vi "SquareFromCenter.vi"(6 "Distance":i32=10, 10 "Top":i32, 11 "Left":i32) -> (0 "Bottom":i32, 1 "Right":i32, 2 "Top 2":i32, 3 "Left 2":i32)   [LabVIEW 2014]
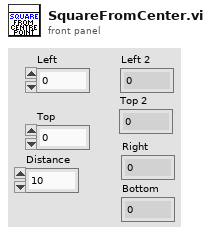
[diagram p1: front panel]
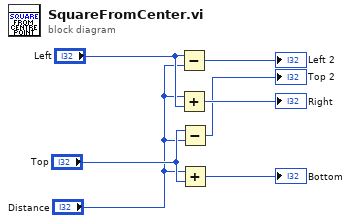
[diagram p0: block diagram]
diagram:
  n1 = Subtract(x="Left", y="Distance") -> (x-y=→"Left 2":i32)
  n2 = Add(x="Distance", y="Left") -> (x+y=→"Right":i32)
  n3 = Subtract(x="Top", y="Distance") -> (x-y=→"Top 2":i32)
  n4 = Add(x="Distance", y="Top") -> (x+y=→"Bottom":i32)
